vi "notch_and_cut.vi"(8 "Parameters":T1={"Order"=0, "Time constant"=0.0, "Detrend mode"=enum."Robust linear", "TD amplitude limit"=inf, "FFT filter"=TRUE, "Notch channels"=[], "LF cutoff"=0, "FD amplitude limit"=0.0}, 11 "In":cdb[](array[numeric])) -> (3 "Out":cdb[](array[numeric]))   [LabVIEW 2014]
uses:
  averaging_filter_params.ctl
  detrend_mode.ctl
panel:
  # "Zero out FFT coefficients according to Notch channels/LF cutoff.  Notching removes carriers from the prediction.  The LF cutoff is useful for distortion because the carrier superposition repeats at a higher rate than the filter order.  Apparent lower frequencies are usually due to non-periodic disturbances."
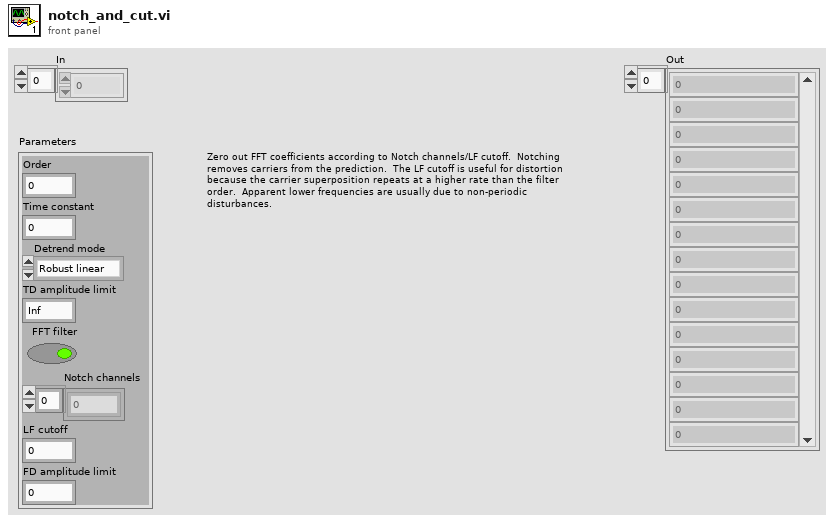
[diagram p1: front panel]
types:
  T1 = typedef "averaging_filter_params.ctl" = cluster{"Order":i32, "Time constant":dbl, "Detrend mode":T2, "TD amplitude limit":dbl, "FFT filter":bool, "Notch channels":i32[], "LF cutoff":i32, "FD amplitude limit":dbl}
  T2 = typedef "detrend_mode.ctl" = enum16{"Zero mean", "Linear", "Robust linear"}
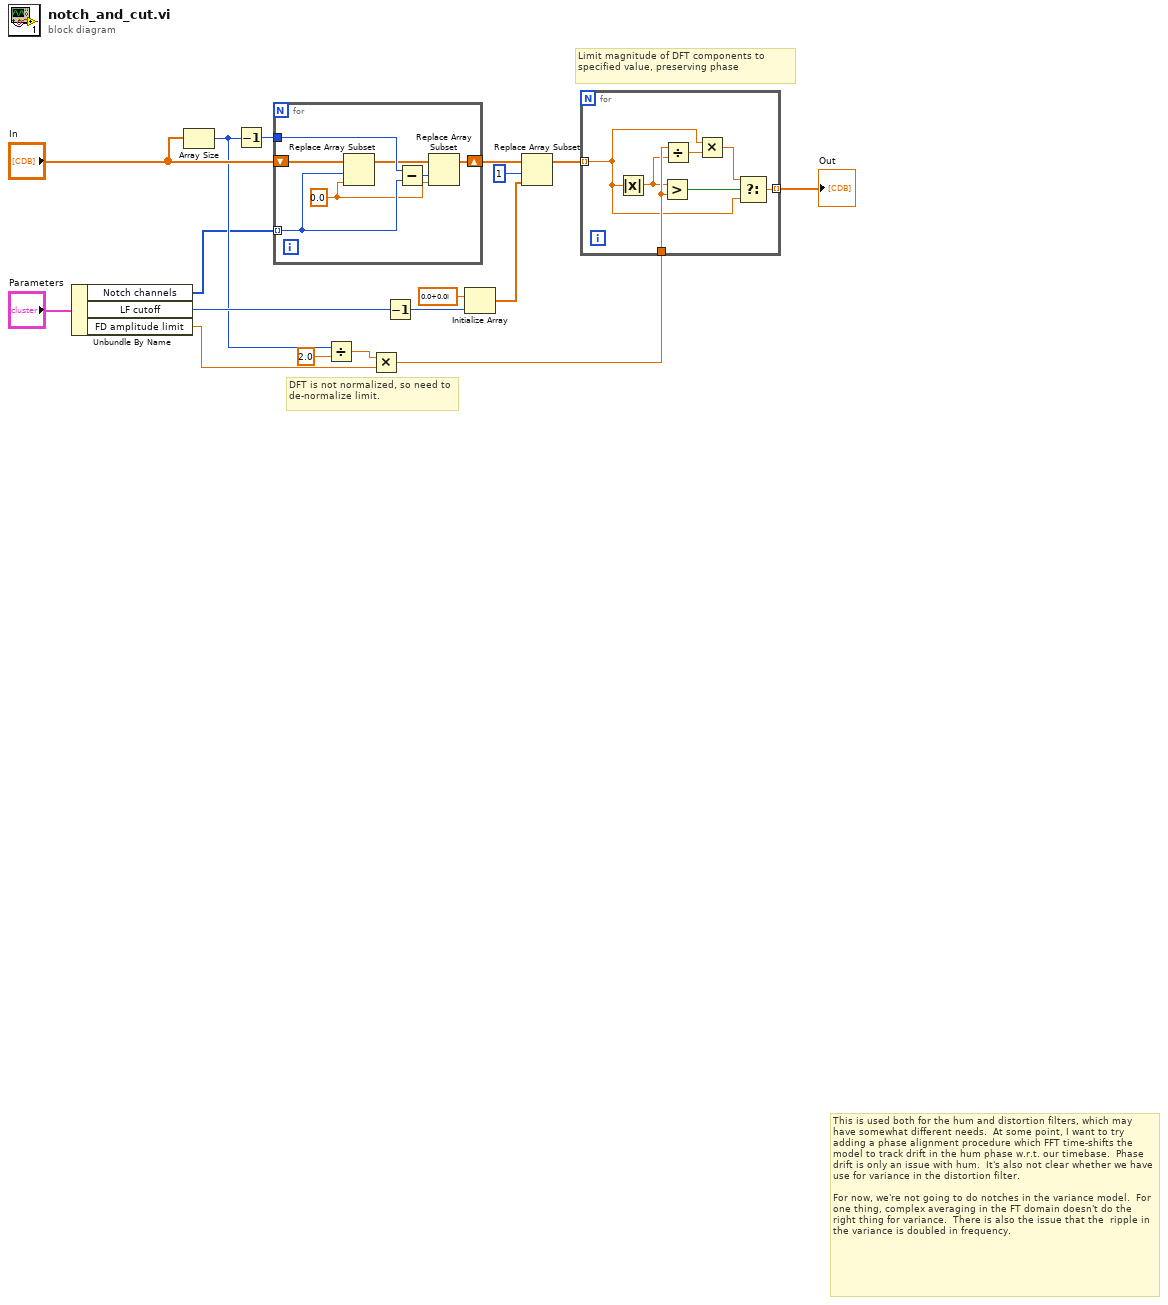
[diagram p0: block diagram]
diagram:
  # "DFT is not normalized, so need to de-normalize limit."
  # "Limit magnitude of DFT components to specified value, preserving phase"
  # "This is used both for the hum and distortion filters, which may have somewhat different needs.  At some point, I want to try adding a phase alignment procedure which FFT time-shifts the model to track drift in the hum phase w.r.t. our timebase.  Phase drift is only an issue with hum.  It's also not clear whether we have use for variance in the distortion filter.\n\nFor now, we're not going to do notches in the variance model.  For one thing, complex averaging in the FT domain doesn't do the right thing for variance.  There is also the issue that the  ripple in the variance is doubled in frequency."
  n1 = Unbundle By Name("Parameters") -> ("Notch channels"=w2:i32[], "LF cutoff"=w9:i32, "FD amplitude limit"=w5:dbl)
  n2 = Array Size(array="In") -> (size(s)=w4:i32)
  n3 = Decrement(x=w4) -> (x-1=w15:i32)
  n4 = for {
    shift-right: [w19] -> w13
    shift-left: "In" -> [w24]
    tunnel: w2 -> [w22] mode=indexing
    tunnel: w15 -> [w23]
    w18 = 0.0
    n5 = Replace Array Subset(array=w24, new element=w18, index=w22) -> (w20:cdb[])
    n6 = Subtract(x=w23, y=w22) -> (x-y=w21:i32)
    n7 = Replace Array Subset(array=w20, new element=w18, index=w21) -> (w19:cdb[])
  }
  n8 = Divide(x=w4, y=2.0 ("x")) -> (x/y=w3:dbl)
  n9 = Multiply(x=w3, y=w5) -> (x*y=w6:dbl)
  n10 = Decrement(x=w9) -> (x-1=w8:i32)
  n11 = Initialize Array(cdb 0.0+0.0i, w8) -> (w12:cdb[])
  n12 = Replace Array Subset(array=w13, new element=w12, index=1) -> (w7:cdb[])
  n13 = for {
    tunnel: w7 -> [w27] mode=indexing
    tunnel: w6 -> [w30]
    tunnel: [w25] -> w16 mode=indexing
    n14 = Absolute Value(x=w27) -> (abs(x)=w29:dbl)
    n15 = Greater?(x=w29, y=w30) -> (0:w31:bool)
    n16 = Divide(x=w30, y=w29) -> (x/y=w28:dbl)
    n17 = Multiply(x=w27, y=w28) -> (x*y=w26:cdb)
    n18 = Select(t=w26, s=w31, f=w27) -> (s? t:f=w25:cdb)
  }
  "Out" <- w16
